vi "Extraccion_datos.vi"() -> ()   [LabVIEW 2017]
uses:
  <vilib>/addons/Biomedical/Controls/Biosignal/Biosignal Spectrum/Biosignal Spectrum.xctl
  <vilib>/addons/Biomedical/Biosignal Measurements/EEG/EEG FFT Spectrum (Waveform).vi
  <vilib>/addons/Biomedical/NI_BMTK_Measurements.lvlib
  <vilib>/addons/Biomedical/NI_BMTK_Controls.lvlib
panel:
  in  "Speed":u32(slide)=100 scale=5.0..100.0
  in  "Stop":bool
  in  "error in (no error)":errorcluster
  out "EEG Spectrum":cluster{"f0":dbl, "df":dbl, "S(f)":dbl[]}(xcontrol)
  out "Beta [%]":dbl format="%#_2f %"
  out "Beta Power":dbl format="%#_2f uV^2"
  out "Alpha [%]":dbl format="%#_2f %"
  out "Theta [%]":dbl format="%#_2f %"
  out "Delta [%]":dbl format="%#_2f %"
  out "Alpha Power":dbl format="%#_2f uV^2"
  out "Theta Power":dbl format="%#_2f uV^2"
  out "Delta Power":dbl format="%#_2f uV^2"
  out "EEG":dynamicdata(graph)
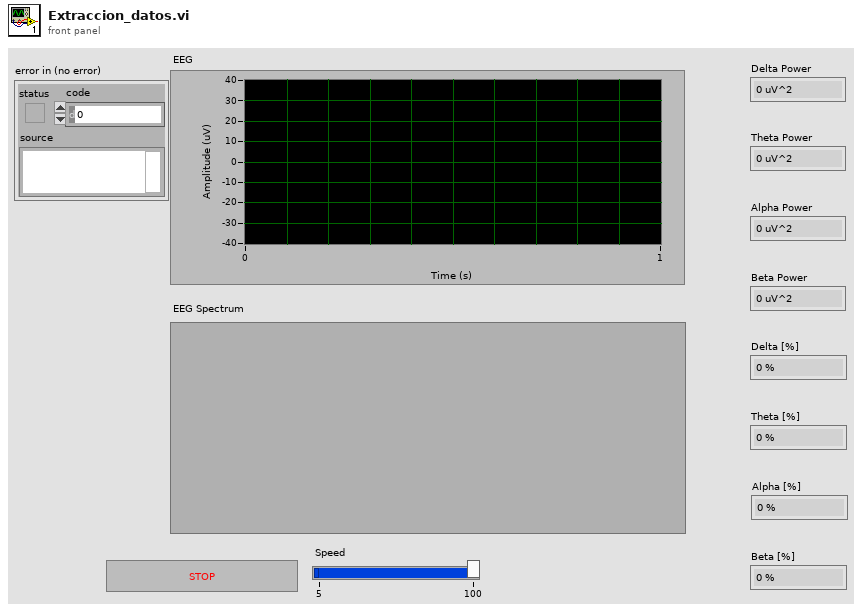
[diagram p1: front panel]
types:
  T1 = enum16{"open", "replace", "create", "open or create", "replace or create", "replace or create with confirmation"}
  T2 = typedef "NI_BMTK_Measurements.lvlib/bmt_EEG Frequency-domain Measures.ctl" = cluster{"delta power":dbl, "theta power":dbl, "alpha power":dbl, "beta power":dbl, "delta [%]":dbl, "theta [%]":dbl, "alpha [%]":dbl, "beta [%]":dbl}
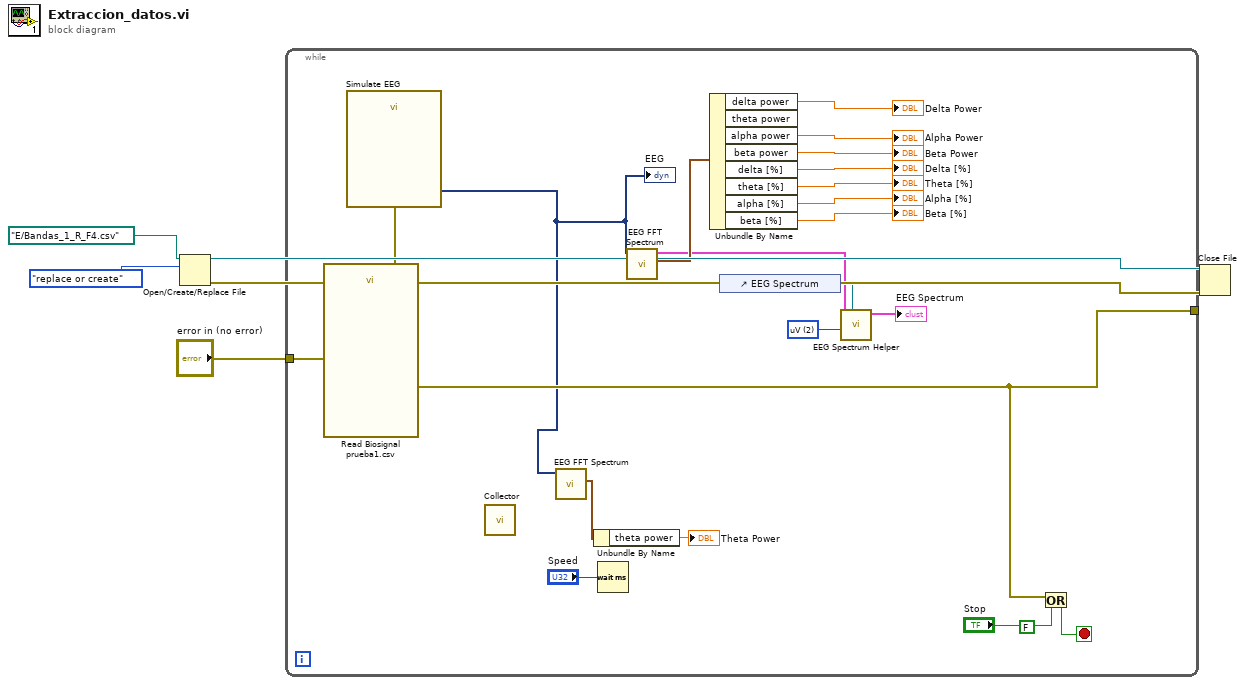
[diagram p0: block diagram]
diagram:
  n1 = Open/Create/Replace File(file path (use dialog)=path "E:/Bandas_1_R_F4.csv" ("edk.dll Path"), operation (0:open)=T1."replace or create") -> (refnum out=w2:refnum<file>, error out=w3:errorcluster)  [unwired: 4 in, 1 out]
  n2 = while {
    tunnel: "error in (no error)" -> [w7]
    tunnel: [w12] -> _
    stop <- w11 stop-if-true
    (unwired) FALSE
    w17 = u16 2 items=["V", "mV", "uV"] ("RR unit")
    n3 = call "Read Biosignal\nprueba1.csv"() -> ("error out"=w12:errorcluster)  [unwired: 11 in, 4 out]
    n4 = call "Simulate EEG"("error in (no error)"=w7) -> ("EEG"=w6:dynamicdata)  [unwired: 9 in, 1 out]
    "EEG" <- w6
    n5 = call "Collector"() -> ()  [unwired: 10 in, 2 out]
    n6 = call-poly <vilib>:"EEG FFT Spectrum.vi"("EEG"=w6) -> ("frequency measurements"=w9:T2)  [unwired: 8 in, 2 out]
    n7 = Unbundle By Name(w9) -> ("theta power"=→"Theta Power":dbl)
    n8 = Wait (ms)(milliseconds to wait="Speed") -> ()  [unwired: 1 out]
    n9 = call-poly <vilib>:"EEG FFT Spectrum.vi"("EEG"=w6) -> ("frequency measurements"=w25:T2, "FFT spectrum"=w14:cluster{"f0":dbl, "df":dbl, "S(f)":dbl[]})  [unwired: 8 in, 1 out]
    n10 = Unbundle By Name(w25) -> ("delta power"=→"Delta Power":dbl, "alpha power"=→"Alpha Power":dbl, "beta power"=→"Beta Power":dbl, "delta [%]"=→"Delta [%]":dbl, "theta [%]"=→"Theta [%]":dbl, "alpha [%]"=→"Alpha [%]":dbl, "beta [%]"=→"Beta [%]":dbl)  [unwired: 1 out]
    n11 = control-ref of="EEG Spectrum"() -> (w16:refnum<vi>)
    n12 = call <vilib>:"EEG Spectrum Helper.vi"("EEG spectrum"=w16, "EEG unit"=w17, "spectrum in"=w14) -> ("spectrum out"=→"EEG Spectrum":cluster{"f0":dbl, "df":dbl, "S(f)":dbl[]})  [unwired: 7 in, 1 out]
    n13 = Or(x=w12, y="Stop") -> (x .or. y?=w11:bool)
  }
  n14 = Close File(refnum=w2, error in=w3) -> ()  [unwired: 2 out]
